vi "fgv_ledmatrix_arduino.vi"(7 "cmd":enum16{"init", "read", "write", "close"}(ring), 8 "error in":errorcluster, 11 "cmd 2":string) -> (0 "error out":errorcluster, 2 "val":bool, 3 "read_buffer":string)   [LabVIEW 2019]
uses:
  Ctrl/cmd_common.ctl
  <vilib>/Instr/_visa.llb/VISA Configure Serial Port (Instr).vi
panel:
  out "send_data":u8[](array[numeric]) format="%x"
  out "cmd out":string
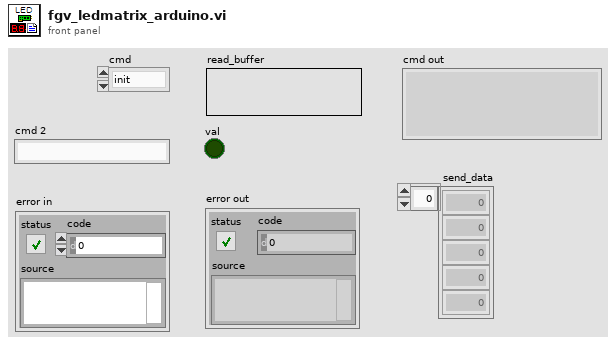
[diagram p1: front panel]
types:
  T1 = typedef "cmd_common.ctl" = enum16{"read", "write"}
  T2 = typedef "ledmatrix_data.ctl" = cluster{"ip":string, "data":string, "Port":refnum<visa-resource-name>, "latlong":string}
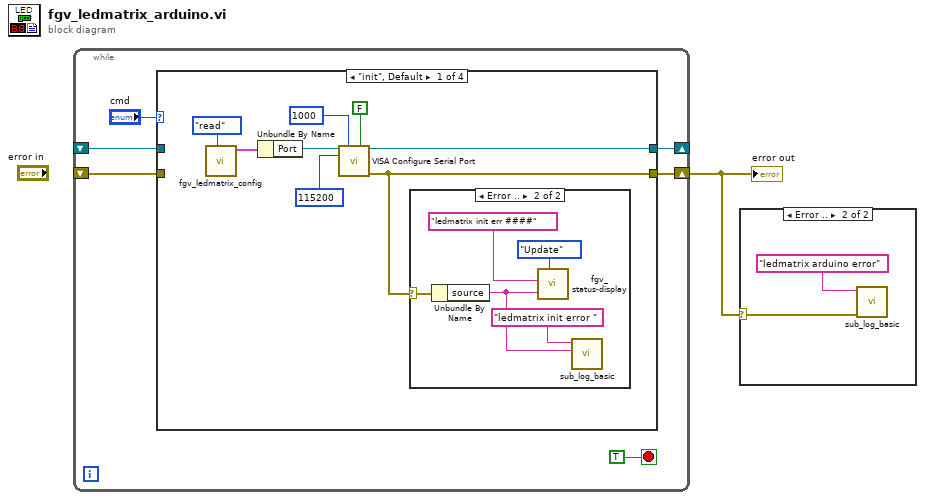
[diagram p0: block diagram]
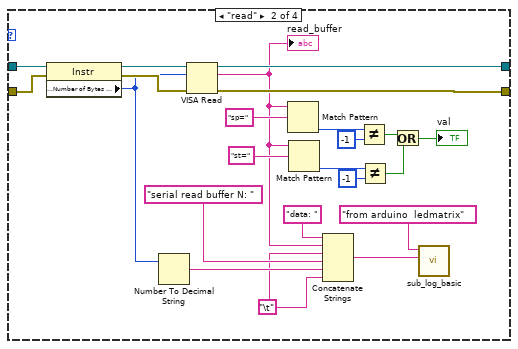
[diagram p4: hidden frame]
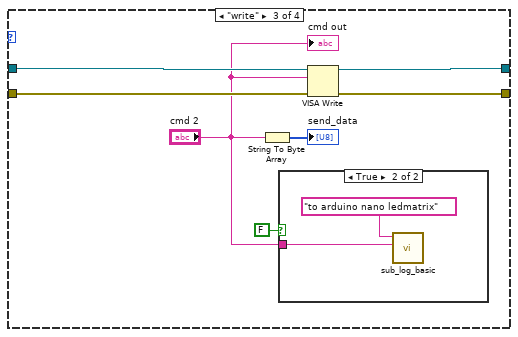
[diagram p5: hidden frame]
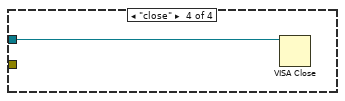
[diagram p7: hidden frame]
diagram:
  n1 = while {
    shift-right: [w5] -> _
    shift-left: _ -> [w3]
    shift-right: [w4] -> w1
    shift-left: _ -> [w2]
    stop <- TRUE stop-if-true
    n2 = case shown="\"init\", Default" "cmd" {
      tunnel: [w14 w41 w48 _] -> w5
      tunnel: [w9 w40 w47 _] -> w4
      tunnel: w3 -> [_ w43 w49 w53]
      tunnel: w2 -> [_ w38 w50 _]
      frame "init", Default {
        n3 = call "fgv_ledmatrix_config.vi"("cmd"=cmd_common."read") -> ("data out"=w11:T2)  [unwired: 10 in]
        n4 = Unbundle By Name(w11) -> ("Port"=w10:refnum<visa-resource-name>)
        n5 = call-poly "VISA Configure Serial Port"("VISA resource name"=w10, "timeout (10sec)"=u32 1000, "Enable Termination\nChar (T)"=FALSE ("Enable Termination\nChar (T)"), "baud rate (9600)"=u32 115200) -> ("VISA resource name out"=w14:refnum<visa-resource-name>, "error out"=w9:errorcluster)  [unwired: 10 in]
        n6 = case shown="Error .." w9 {
          selector: w9 -> [_ w18]
          frame No Error {
          }
          frame Error {
            n7 = Unbundle By Name(w18) -> ("source"=w16:string)
            n8 = call "fgv_status-display.vi"("Mode"=enum16{"Initial", "Update", "Clear"}."Update", "detail"=w16, "title"="ledmatrix init err ####" ("String in")) -> ()  [unwired: 8 in, 1 out]
            n9 = call "sub_log_basic.vi"("desc"=w16, "Title"="ledmatrix init error ") -> ()  [unwired: 9 in, 1 out]
          }
        }
      }
      frame "read" {
        w23 = "\t"
        n10 = property class="Instr"(reference=w43, error in=w38) -> (reference out=w42:refnum<visa-resource-name>, error out=w39:errorcluster, "Serial Settings:Number of Bytes at Serial Port"=w27:u32)
        n11 = Number To Decimal String(number=w27) -> (decimal integer string=w25:string)  [unwired: 1 in]
        n12 = VISA Read(VISA resource name=w42, byte count=w27, error in (no error)=w39) -> (VISA resource name out=w41:refnum<visa-resource-name>, read buffer=w21:string, error out=w40:errorcluster)  [unwired: 1 out]
        "read_buffer" <- w21
        n13 = Match Pattern(string=w21, regular expression="sp=") -> (offset past match=w36:i32)  [unwired: 1 in, 3 out]
        n14 = Match Pattern(string=w21, regular expression="st=") -> (offset past match=w33:i32)  [unwired: 1 in, 3 out]
        n15 = Concatenate Strings("data: " ("문자열"), w21, w23, "serial read buffer N: " ("문자열"), w25, w23) -> (w22:string)
        n16 = Not Equal?(x=w36, y=-1) -> (x != y?=w31:bool)
        n17 = Not Equal?(x=w33, y=-1) -> (x != y?=w32:bool)
        n18 = Or(x=w31, y=w32) -> (x .or. y?=→"val":bool)
        n19 = call "sub_log_basic.vi"("desc"=w22, "Title"="from arduino  ledmatrix") -> ()  [unwired: 9 in, 1 out]
      }
      frame "write" {
        n20 = String To Byte Array(string="cmd 2") -> (unsigned byte array=→"send_data":u8[])
        n21 = case shown="True" FALSE {
          tunnel: "cmd 2" -> [_ w51]
          frame False {
          }
          frame True {
            n22 = call "sub_log_basic.vi"("desc"=w51, "Title"="to arduino nano ledmatrix") -> ()  [unwired: 9 in, 1 out]
          }
        }
        n23 = VISA Write(VISA resource name=w49, write buffer="cmd 2", error in (no error)=w50) -> (VISA resource name out=w48:refnum<visa-resource-name>, error out=w47:errorcluster)  [unwired: 1 out]
        "cmd out" <- "cmd 2"
      }
      frame "close" {
        n24 = VISA Close(VISA resource name=w53) -> ()  [unwired: 1 in, 1 out]
      }
    }
  }
  "error out" <- w1
  n25 = case shown="Error .." w1 {
    selector: w1 -> [_ w54]
    frame No Error {
    }
    frame Error {
      n26 = call "sub_log_basic.vi"("error in"=w54, "Title"="ledmatrix arduino error") -> ()  [unwired: 9 in, 1 out]
    }
  }
